vi "Generate Random GB of Size 2015-01-08.vi"() -> ()   [LabVIEW 2010]
uses:
  <vilib>/Utility/file.llb/Write To Spreadsheet File (string).vi
panel:
  out "GBs to Make":cluster{dbl[], dbl[], "Parameter":dbl, dbl[]}[](array[cluster])
  out "# Created":i32
  out "Grain Boundary Definition":T1={"Grain 1 Orientation"=[1.0, 0.8858401549498205, 0.0], "Grain 2 Orientation"=[1.0, 0.3745791306245927, 0.0], "Twist Angle (Deg)"=39.42112887005932, "Translation Vector"=[0.0, 0.0, 0.0]}
  out "Current Index":i32=165102
  out "Status":string="Within range!\nNow creating...\nChecking expected size\nRolling dice...\n"
  in  "Make Random GBs Tab":T2(tab)
  in  "# of Points, Translation":i32
  in  "# of Points, Angle":i32
  in  "# of Points, G2":i32
  in  "Grain 2 or Misorientation Axis":T3={"h, min"=1.0, "h, max"=1.0, "k, min"=0.0, "k, max"=1.0, "l, min"=0.0, "l, max"=1.0} caption="Grain 2 Orientation" {"h, min" format="%#_4f"; "h, max" format="%#_4f"; "k, min" format="%#_4f"; "k, max" format="%#_4f"; "l, min" format="%#_4f"; "l, max" format="%#_4f"}
  in  "Force h>k>l ?":bool=TRUE
  in  "Grain DoF Style":enum32{"Interface-Plane", "Misorientation"}(radio)
  in  "Creation Style":enum32{"Random", "Sequential"}(radio)
  in  "Grain 1 Orientation":T3={"h, min"=1.0, "h, max"=1.0, "k, min"=0.0, "k, max"=1.0, "l, min"=0.0, "l, max"=1.0} {"h, min" format="%#_4f"; "h, max" format="%#_4f"; "k, min" format="%#_4f"; "k, max" format="%#_4f"; "l, min" format="%#_4f"; "l, max" format="%#_4f"}
  in  "Angle Min":dbl caption="Twist Angle"
  in  "Angle Max":dbl=64.0 caption="Max"
  in  "Nearest Integers?":bool
  in  "# to Make":i32
  in  "Translation":T4={"T_x min"=0.0, "T_x max"=3.3, "T_y min"=0.0, "T_y max"=3.3, "T_z min"=0.0, "T_z max"=3.3} {"T_x min" format="%#_4f"; "T_x max" format="%#_4f"; "T_y min" format="%#_4f"; "T_y max" format="%#_4f"; "T_z min" format="%#_4f"; "T_z max" format="%#_4f"}
  in  "# of Points, G1":i32
  out "# of total points":i32
  in  "Max # of Atoms":i32=500
  in  "Require STEM Viewable?":bool
  in  "Number of integers to search":i32=50
  in  "Co-incident Tolerance":dbl=0.01
  in  "Grain Growth and Geometry":T5={"Min Grain Length (A)"=5.0, "Min Angle from GB plane"=0.0, "GB Overlap Length (A)"=0.0}
  in  "Min Seperation Distance (A)":dbl=2.0
  in  "Edge Duplication Range":dbl=3.0
  out "Expected # of atoms":i32=472
  out "# of atoms":i32=2541
  in  "Output Directory":path=path "D:/Ab-initio/RAGB3"
  out "Last Creation Time":T6={"Time to create primitives"=1, "Time to Grow to Box"=5932, "Time to find subset"=6894, "Time to Cleanup"=0}
  out "Structures / Minute":dbl
  in  "Stop Making GBs":bool
  in  "Start Making GBs":bool
  in  "Making GBs":bool
  in  "Conventional Unit Cell":T7={"Structure Name"="CdTe", "Lattice vector a"=[6.615785553057252, 0.0, 0.0], "Lattice vector b"=[0.0, 6.615785553057252, 0.0], "Lattice vector c"=[0.0, 0.0, 6.615785553057252], "Atoms Array"=[{"Atom Name"="Cd", "Positions (Direct)"=[[0.0, 0.0, 0.0], [0.0, 0.5, 0.5], [0.5, 0.0, 0.5], [0.5, 0.5, 0.0]], "Positions (Cartesian)"=[[0.0, 0.0, 0.0], [0.0, 3.307892776528626, 3.307892776528626], [3.307892776528626, 0.0, 3.307892776528626], [3.307892776528626, 3.307892776528626, 0.0]]}, {"Atom Name"="Te", "Positions (Direct)"=[[0.25, 0.25, 0.25], [0.75, 0.75, 0.25], [0.75, 0.25, 0.75], [0.25, 0.75, 0.75]], "Positions (Cartesian)"=[[1.653946388264313, 1.653946388264313, 1.653946388264313], [4.96183916479294, 4.96183916479294, 1.653946388264313], [4.96183916479294, 1.653946388264313, 4.96183916479294], [1.653946388264313, 4.96183916479294, 4.96183916479294]]}], "# of atoms"=8}
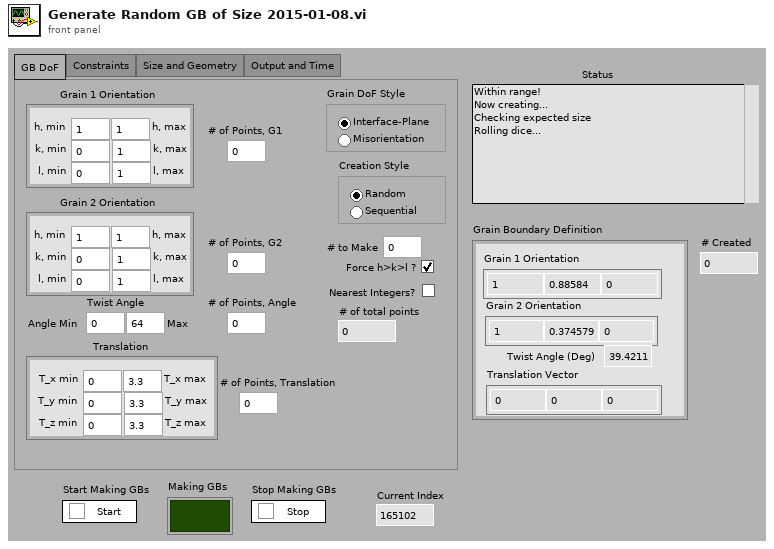
[diagram p1: front panel]
types:
  T1 = cluster{"Grain 1 Orientation":dbl[], "Grain 2 Orientation":dbl[], "Twist Angle (Deg)":dbl, "Translation Vector":dbl[]}
  T2 = enum32{"GB DoF", "Constraints", "Size and Geometry", "Output and Time"}
  T3 = cluster{"h, min":dbl, "h, max":dbl, "k, min":dbl, "k, max":dbl, "l, min":dbl, "l, max":dbl}
  T4 = cluster{"T_x min":dbl, "T_x max":dbl, "T_y min":dbl, "T_y max":dbl, "T_z min":dbl, "T_z max":dbl}
  T5 = cluster{"Min Grain Length (A)":dbl, "Min Angle from GB plane":dbl, "GB Overlap Length (A)":dbl}
  T6 = cluster{"Time to create primitives":u32, "Time to Grow to Box":u32, "Time to find subset":u32, "Time to Cleanup":u32}
  T7 = cluster{"Structure Name":string, "Lattice vector a":dbl[], "Lattice vector b":dbl[], "Lattice vector c":dbl[], "Atoms Array":cluster{"Atom Name":string, "Positions (Direct)":dbl[][], "Positions (Cartesian)":dbl[][]}[], "# of atoms":i32}
  T8 = cluster{dbl[], "Grain 2 Orientation":dbl[], "Twist Angle (Deg)":dbl, dbl[]}
  T9 = cluster{dbl[], "Grain 2 Orientation":dbl[], "Twist Angle (Deg)":dbl}
  T10 = typedef "NI_Matrix.lvlib/RealMatrix.ctl" = dbl[][]
  T11 = cluster{"Misorientation Angle":dbl, "Misorientation Axis, o":dbl[], "Misorientation Matrix":T10}
  T12 = cluster{"h, min":dbl, "h, max":dbl, "# of Points, G1":i32}
  T13 = cluster{"k, min":dbl, "k, max":dbl, "# of Points, G1":i32}
  T14 = cluster{"l, min":dbl, "l, max":dbl, "# of Points, G1":i32}
  T15 = cluster{"h, min":dbl, "h, max":dbl, "# of Points, G2":i32}
  T16 = cluster{"k, min":dbl, "k, max":dbl, "# of Points, G2":i32}
  T17 = cluster{"l, min":dbl, "l, max":dbl, "# of Points, G2":i32}
  T18 = cluster{"Angle Min":dbl, "Angle Max":dbl, "# of Points, Angle":i32}
  T19 = cluster{"T_x min":dbl, "T_x max":dbl, "# of Points, Translation":i32}
  T20 = cluster{"T_y min":dbl, "T_y max":dbl, "# of Points, Translation":i32}
  T21 = cluster{"T_z min":dbl, "T_z max":dbl, "# of Points, Translation":i32}
  T22 = cluster{"T_z min":dbl, "T_z max":dbl, "# of Points, Translation":i32}[]
  T23 = cluster{"T_z min":dbl, "T_z max":dbl, "# of Points, Translation":i32, "Style":enum16{"Linear Step", "Linear Pts", "Log Pts"}, string}
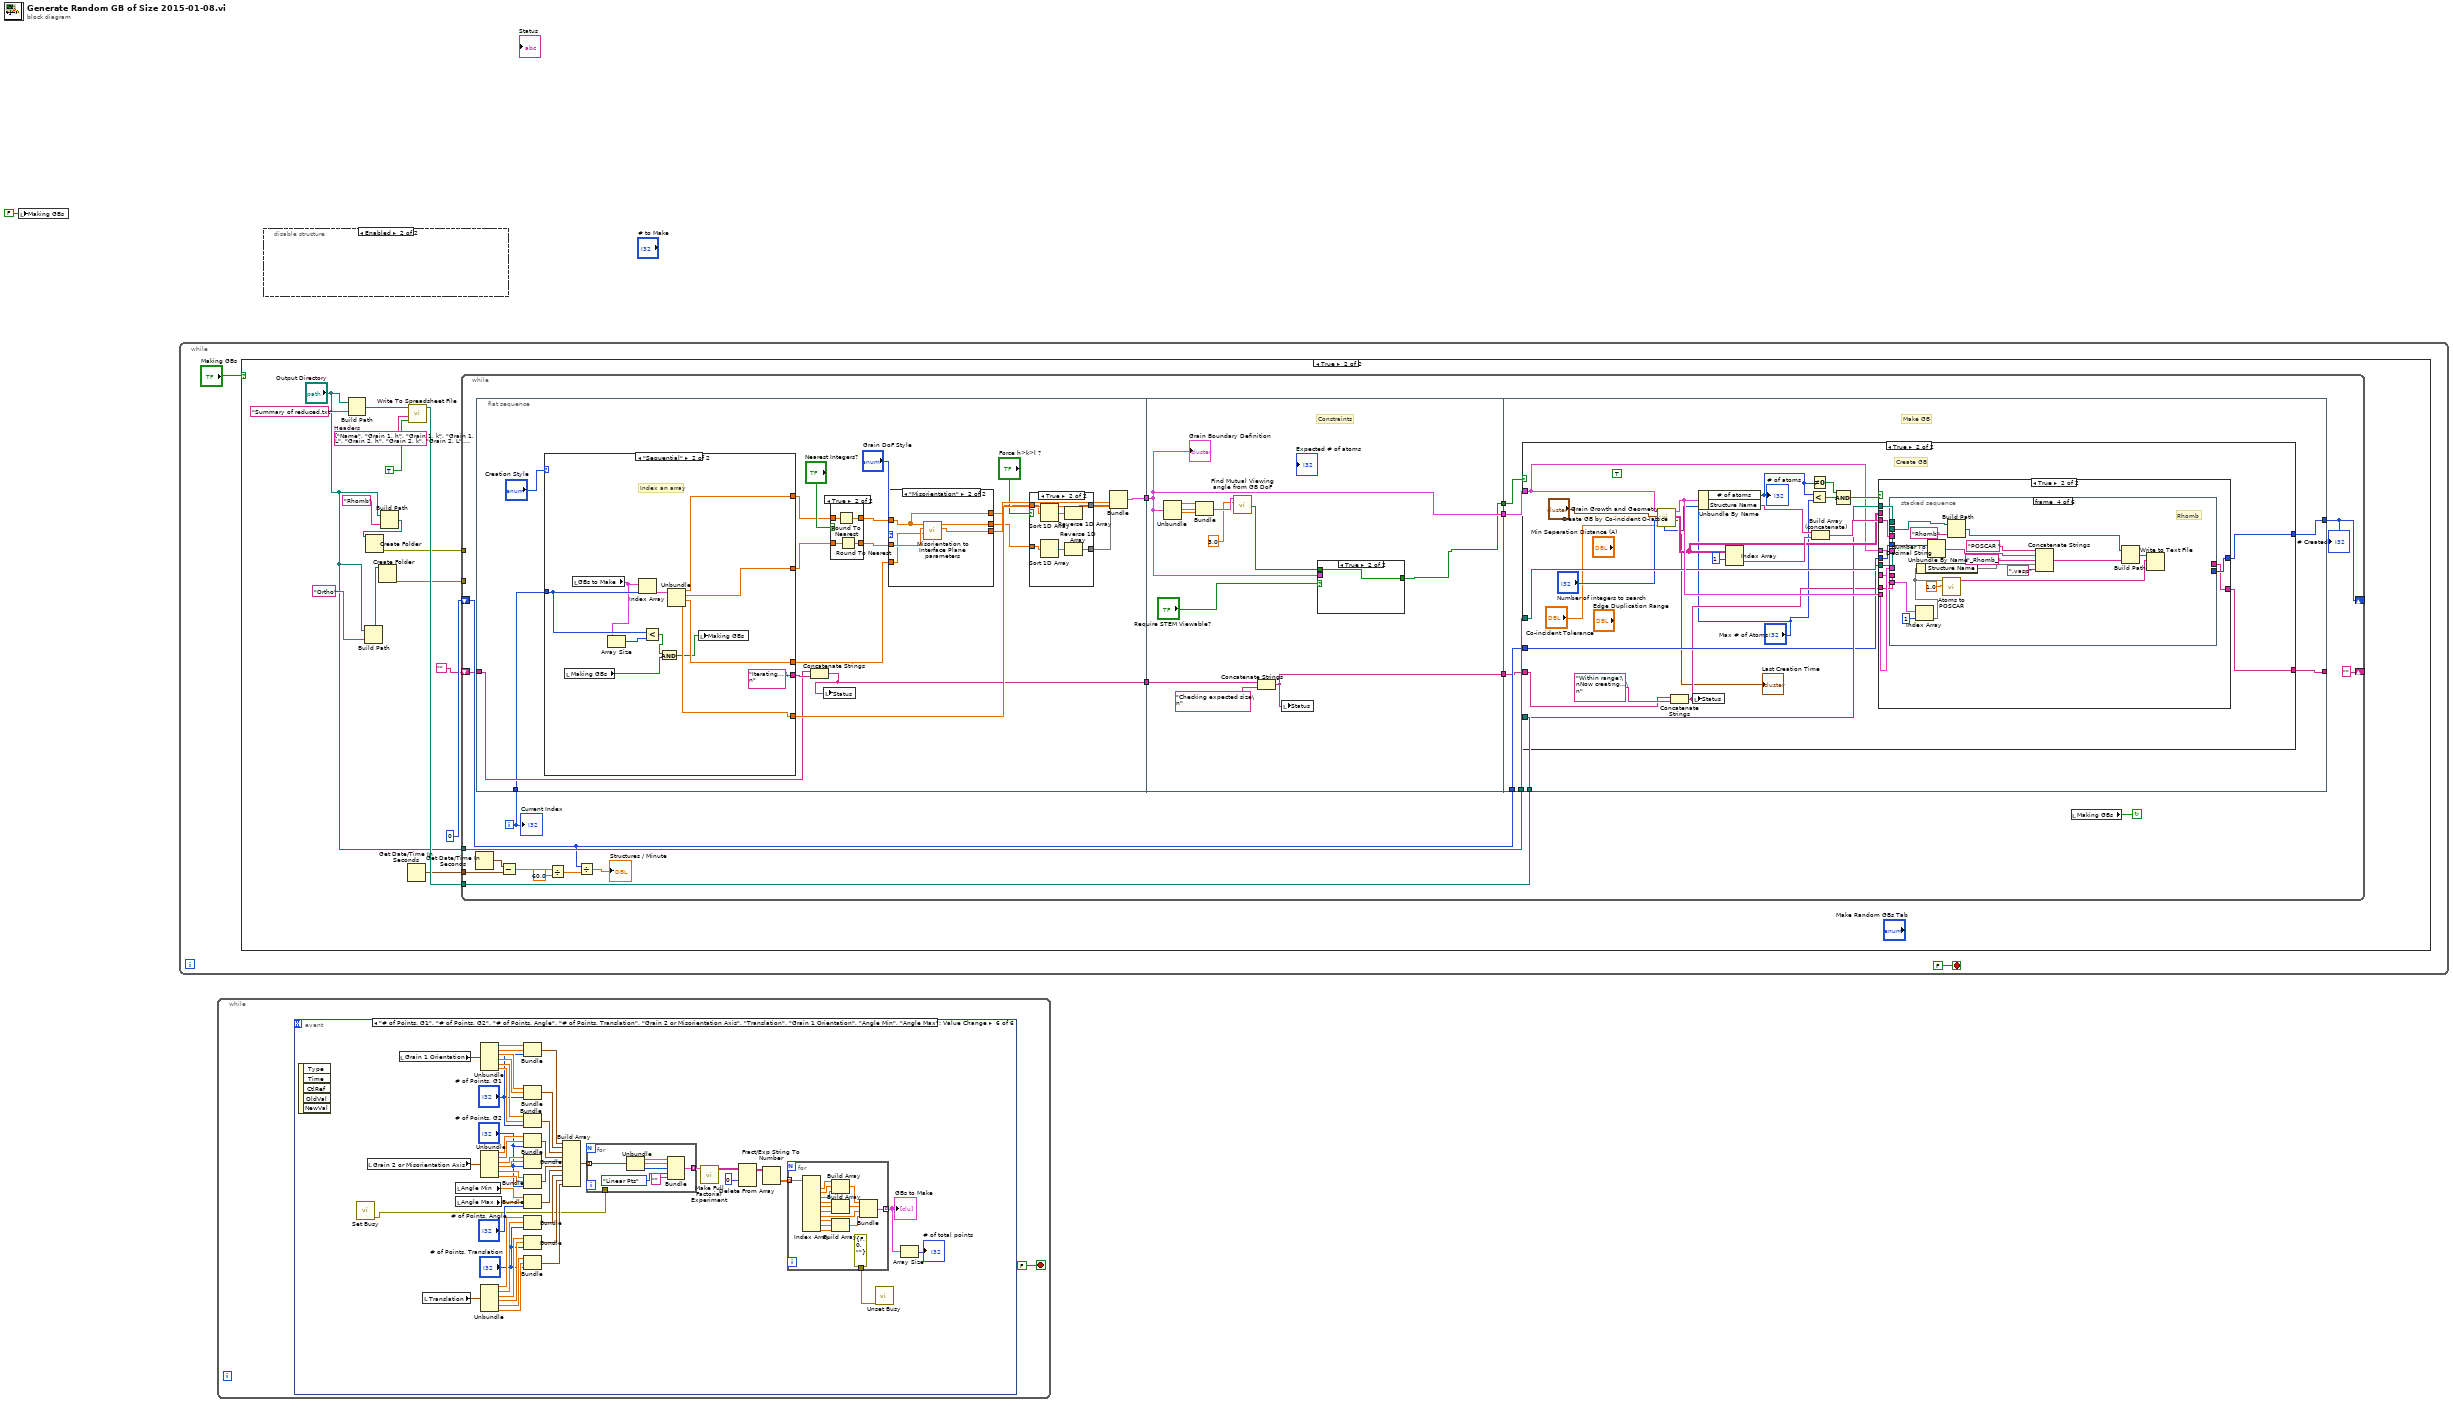
[diagram p0: block diagram]
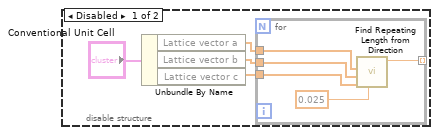
[diagram p2: hidden frame]
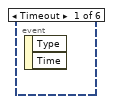
[diagram p3: hidden frame]
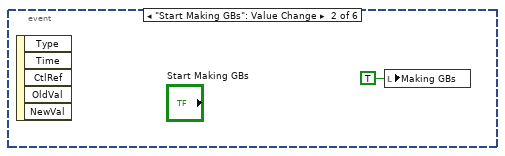
[diagram p4: hidden frame]
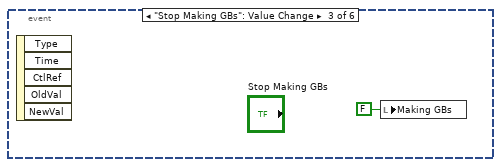
[diagram p5: hidden frame]
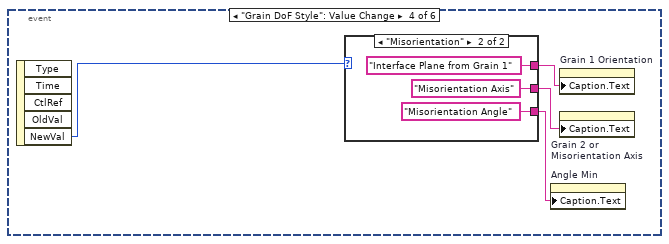
[diagram p6: hidden frame]
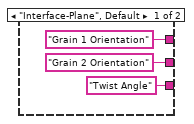
[diagram p7: hidden frame]
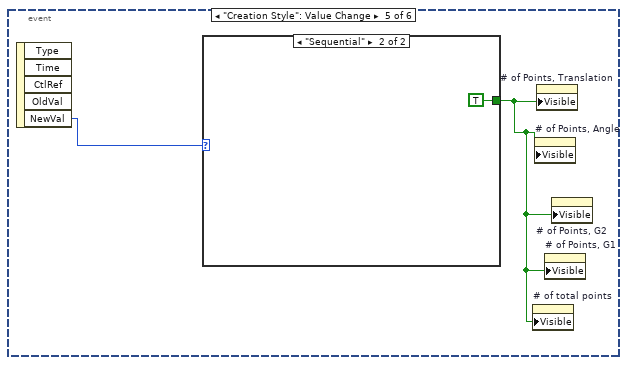
[diagram p8: hidden frame]
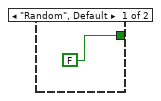
[diagram p9: hidden frame]
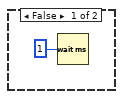
[diagram p10: hidden frame]
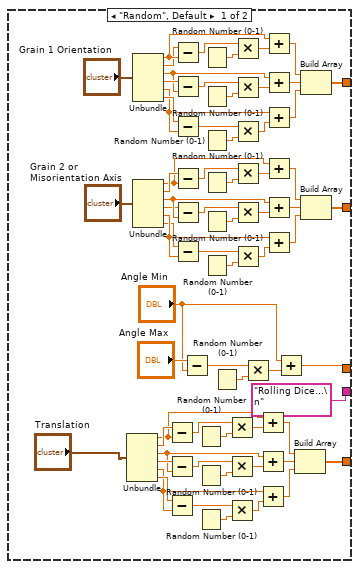
[diagram p14: hidden frame]
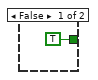
[diagram p15: hidden frame]
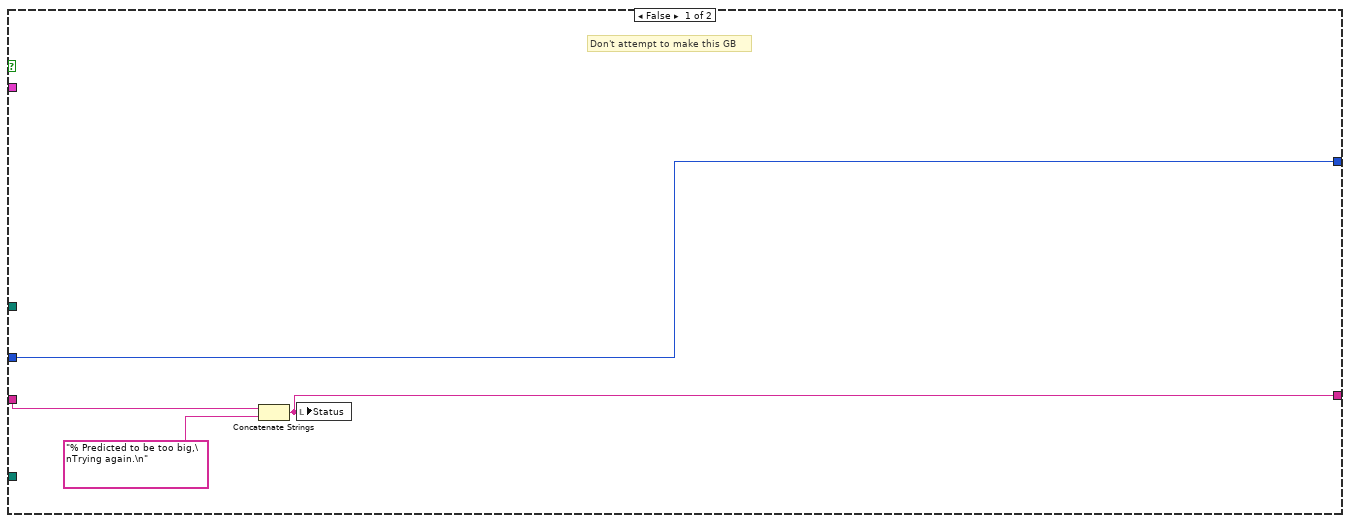
[diagram p16: hidden frame]
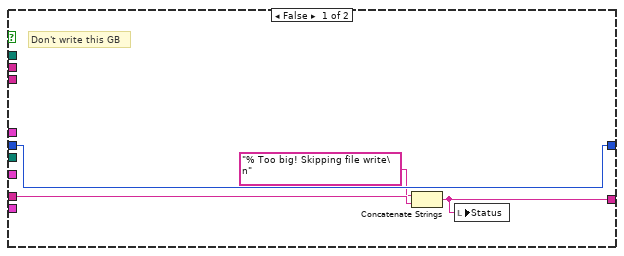
[diagram p17: hidden frame]
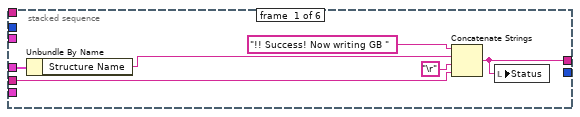
[diagram p18: hidden frame]
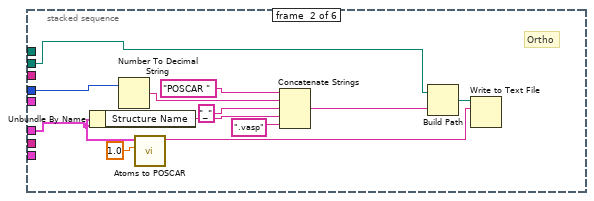
[diagram p19: hidden frame]
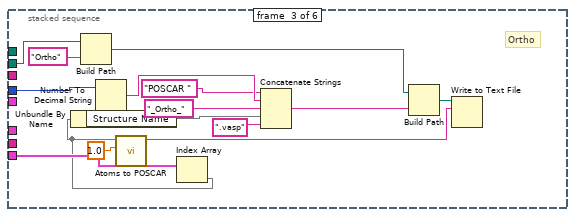
[diagram p20: hidden frame]
diagram:
  n1 = local write "Making GBs"(FALSE ("Making GBs")) -> ()
  n2 = while {
    stop <- FALSE stop-if-true
    n3 = case shown="True" "Making GBs" {
      frame False {
        n4 = Wait (ms)(milliseconds to wait=u32 1) -> ()  [unwired: 1 out]
      }
      frame True {
        w16 = string[] ["Name", "Grain 1, h", "Grain 1, k", "Grain 1, L", "Grain 2, h", "Grain 2, k", "Grain 2, L", "Twist Angle (Deg)", "Translation Tx", "Translation Ty", "Translation Tz", "Tilt Angle (Deg)", "Viewing Angle, h", "Viewing Angle, k", "Viewing Angle, L", "Grain 1 Length (factor)", "Grain 2 Length (factor", "Max Grain Height (A)", "Max Grain Width (A)", "Grain 1 Start", "Overlap Region (A)", "Reduction Slab X", "Reduction Slab Y", "Reduction Tolerance (A)", "Min Atomic Separation Distance", "Edge Duplication Range", "# of Atoms", "STEM Direction,h", "STEM Direction,k", "STEM Direction,l", "Grain 1, [h]", "Grain 1, [k]", "Grain 1, [L]", "Grain 2, [h]", "Grain 2, [k]", "Grain 2, [L]", "Misorientaton Angle (Deg)", "Misorientation Axis, h", "Misorientation Axis, k", "Misorientation Axis, l"]  # Headers
        n5 = Build Path(base path="Output Directory", name or relative path="Summary of reduced.txt") -> (appended path=w17:path)
        n6 = Build Path(base path="Output Directory", name or relative path="Ortho") -> (appended path=w8:path)
        n7 = Create Folder(path (use dialog)=w8) -> (error out=w6:errorcluster)  [unwired: 2 in, 2 out]
        n8 = Build Path(base path="Output Directory", name or relative path="Rhomb") -> (appended path=w10:path)
        n9 = Create Folder(path (use dialog)=w10) -> (error out=w7:errorcluster)  [unwired: 2 in, 2 out]
        n10 = Get Date/Time In Seconds() -> (seconds since 1Jan1904=w12:timestamp)
        n11 = call-poly <vilib>:"Write To Spreadsheet File.vi"("append to file? (new file:F)"=TRUE, "1D data"=w16, "file path (dialog if empty)"=w17) -> ("new file path (Not A Path if cancelled)"=w14:path)  [unwired: 5 in]
        n12 = while {
          shift-right: [w28] -> _
          shift-left: 0 -> [w29]
          tunnel: w12 -> [w35]
          tunnel: "Output Directory" -> [w31]
          tunnel: w14 -> [w30]
          shift-right: [""] -> _
          shift-left: "" -> [w27]
          tunnel: w7 -> [_]
          tunnel: w6 -> [_]
          i -> [w20]
          stop <- w25 continue-if-true
          n13 = Get Date/Time In Seconds() -> (seconds since 1Jan1904=w23:timestamp)
          n14 = flat-sequence {
            tunnel: w27 -> [w40]
            tunnel: [w43] -> w22
            tunnel: [w41] -> w21
            tunnel: w20 -> [w39]
            tunnel: [w168] -> w33
            tunnel: [w160] -> w32
            tunnel: [w170] -> w26
            tunnel: w22 -> [w168]
            tunnel: w21 -> [w163]
            tunnel: w33 -> [w177]
            tunnel: w32 -> [w181]
            tunnel: w31 -> [w180]
            tunnel: w30 -> [w179]
            tunnel: w29 -> [w178]
            tunnel: [w176] -> w28
            tunnel: w26 -> [w175]
            tunnel: [w174] -> _
            frame #0 {
              n15 = case shown="\"Sequential\"" "Creation Style" {
                tunnel: [w110 w157] -> w45
                tunnel: [w109 w156] -> w46
                tunnel: [w103 w155] -> w51
                tunnel: [w84 w154] -> w58
                tunnel: ["Rolling Dice...\n" ("string") "Iterating... \n" ("string")] -> w42
                tunnel: w39 -> [_ w153]
                frame "Random", Default {
                  n16 = Unbundle("Translation") -> ("T_x min"=w82:dbl, "T_x max"=w86:dbl, "T_y min"=w93:dbl, "T_y max"=w94:dbl, "T_z min"=w95:dbl, "T_z max"=w96:dbl)
                  n17 = Unbundle("Grain 1 Orientation") -> ("h, min"=w136:dbl, "h, max"=w133:dbl, "k, min"=w141:dbl, "k, max"=w142:dbl, "l, min"=w143:dbl, "l, max"=w144:dbl)
                  n18 = Unbundle("Grain 2 or Misorientation Axis") -> ("h, min"=w83:dbl, "h, max"=w131:dbl, "k, min"=w124:dbl, "k, max"=w123:dbl, "l, min"=w122:dbl, "l, max"=w121:dbl)
                  n19 = Subtract(x=w86, y=w82) -> (x-y=w87:dbl)
                  n20 = Subtract(x=w94, y=w93) -> (x-y=w90:dbl)
                  n21 = Subtract(x=w96, y=w95) -> (x-y=w91:dbl)
                  n22 = Subtract(x=w133, y=w136) -> (x-y=w134:dbl)
                  n23 = Subtract(x=w142, y=w141) -> (x-y=w138:dbl)
                  n24 = Subtract(x=w144, y=w143) -> (x-y=w139:dbl)
                  n25 = Subtract(x=w131, y=w83) -> (x-y=w130:dbl)
                  n26 = Subtract(x=w123, y=w124) -> (x-y=w127:dbl)
                  n27 = Subtract(x=w121, y=w122) -> (x-y=w126:dbl)
                  n28 = Subtract(x="Angle Max", y="Angle Min") -> (x-y=w106:dbl)
                  n29 = Random Number (0-1)() -> (number: 0 to 1=w97:dbl)
                  n30 = Random Number (0-1)() -> (number: 0 to 1=w98:dbl)
                  n31 = Random Number (0-1)() -> (number: 0 to 1=w99:dbl)
                  n32 = Random Number (0-1)() -> (number: 0 to 1=w145:dbl)
                  n33 = Random Number (0-1)() -> (number: 0 to 1=w146:dbl)
                  n34 = Random Number (0-1)() -> (number: 0 to 1=w147:dbl)
                  n35 = Random Number (0-1)() -> (number: 0 to 1=w120:dbl)
                  n36 = Random Number (0-1)() -> (number: 0 to 1=w119:dbl)
                  n37 = Random Number (0-1)() -> (number: 0 to 1=w118:dbl)
                  n38 = Random Number (0-1)() -> (number: 0 to 1=w108:dbl)
                  n39 = Multiply(x=w87, y=w97) -> (x*y=w88:dbl)
                  n40 = Multiply(x=w90, y=w98) -> (x*y=w89:dbl)
                  n41 = Multiply(x=w91, y=w99) -> (x*y=w92:dbl)
                  n42 = Multiply(x=w134, y=w145) -> (x*y=w135:dbl)
                  n43 = Multiply(x=w138, y=w146) -> (x*y=w137:dbl)
                  n44 = Multiply(x=w139, y=w147) -> (x*y=w140:dbl)
                  n45 = Multiply(x=w130, y=w120) -> (x*y=w129:dbl)
                  n46 = Multiply(x=w127, y=w119) -> (x*y=w128:dbl)
                  n47 = Multiply(x=w126, y=w118) -> (x*y=w125:dbl)
                  n48 = Multiply(x=w106, y=w108) -> (x*y=w107:dbl)
                  n49 = Add(x=w82, y=w88) -> (x+y=w100:dbl)
                  n50 = Add(x=w93, y=w89) -> (x+y=w101:dbl)
                  n51 = Add(x=w95, y=w92) -> (x+y=w102:dbl)
                  n52 = Add(x=w136, y=w135) -> (x+y=w116:dbl)
                  n53 = Add(x=w141, y=w137) -> (x+y=w115:dbl)
                  n54 = Add(x=w143, y=w140) -> (x+y=w114:dbl)
                  n55 = Add(x=w83, y=w129) -> (x+y=w113:dbl)
                  n56 = Add(x=w124, y=w128) -> (x+y=w112:dbl)
                  n57 = Add(x=w122, y=w125) -> (x+y=w111:dbl)
                  n58 = Add(x="Angle Min", y=w107) -> (x+y=w103:dbl)
                  n59 = Build Array(w100, w101, w102) -> (w84:dbl[])
                  n60 = Build Array(w116, w115, w114) -> (w110:dbl[])
                  n61 = Build Array(w113, w112, w111) -> (w109:dbl[])
                }
                frame "Sequential" {
                  # "Index an array"
                  n62 = local read "Making GBs"() -> (w149:bool)
                  n63 = local read "GBs to Make"() -> (w152:cluster{dbl[], dbl[], "Parameter":dbl, dbl[]}[])
                  n64 = Array Size(array=w152) -> (size(s)=w151:i32)
                  n65 = Index Array(array=w152, index=w153) -> (element=w158:cluster{dbl[], dbl[], "Parameter":dbl, dbl[]})
                  n66 = Less?(x=w153, y=w151) -> (x < y?=w150:bool)
                  n67 = And(x=w150, y=w149) -> (x .and. y?=w148:bool)
                  n68 = Unbundle(w158) -> (w157:dbl[], w156:dbl[], "Parameter"=w155:dbl, w154:dbl[])
                  n69 = local write "Making GBs"(w148) -> ()
                }
              }
              n70 = Concatenate Strings(w40, w42) -> (w41:string)
              n71 = local write "Status"(w41) -> ()
              n72 = case shown="True" "Nearest Integers?" {
                tunnel: [w75 w80] -> w50
                tunnel: [w76 w79] -> w49
                tunnel: w45 -> [w76 w78]
                tunnel: w46 -> [w75 w77]
                frame False {
                }
                frame True {
                  n73 = Round To Nearest(number=w78) -> (nearest integer value=w79:dbl[])
                  n74 = Round To Nearest(number=w77) -> (nearest integer value=w80:dbl[])
                }
              }
              n75 = case shown="\"Misorientation\"" "Grain DoF Style" {
                tunnel: w49 -> [w69 w71]
                tunnel: w50 -> [w68 w74]
                tunnel: w51 -> [w67 w73]
                tunnel: [w68 w72] -> w54
                tunnel: [w69 w71] -> w52
                tunnel: [w67 w70] -> w57
                frame "Interface-Plane", Default {
                }
                frame "Misorientation" {
                  n76 = call "Misorientation to Interface Plane parameters.vi"("Misorientation Angle"=w73, "Misorientation Axis, o"=w74, "Grain 1 Orientation"=w71) -> ("Twist Angle (Deg)"=w70:dbl, "Grain 2 Orientation"=w72:dbl[])  [unwired: 5 in, 2 out]
                }
              }
              n77 = case shown="True" "Force h>k>l ?" {
                tunnel: [w60 w64] -> w55
                tunnel: w52 -> [w60 w66]
                tunnel: w54 -> [w59 w62]
                tunnel: [w59 w61] -> w56
                frame False {
                }
                frame True {
                  n78 = Sort 1D Array(array=w66) -> (sorted array=w65:dbl[])
                  n79 = Sort 1D Array(array=w62) -> (sorted array=w63:dbl[])
                  n80 = Reverse 1D Array(array=w65) -> (reversed array=w64:dbl[])
                  n81 = Reverse 1D Array(array=w63) -> (reversed array=w61:dbl[])
                }
              }
              n82 = Bundle(w55, "Grain 2 Orientation"=w56, "Twist Angle (Deg)"=w57, w58) -> (w43:T8)  [unwired: 1 in]
            }
            frame #1 {
              # "Constraints"
              n83 = Unbundle(w168) -> (w167:dbl[], "Grain 2 Orientation"=w166:dbl[], "Twist Angle (Deg)"=w165:dbl)  [unwired: 1 out]
              n84 = Bundle(w167, "Grain 2 Orientation"=w166, "Twist Angle (Deg)"=w165) -> (w164:T9)  [unwired: 1 in]
              n85 = call "Find Mutual Viewing angle from GB DoF.vi"("Viewing Angle Tolerance (Deg)"=3.0 ("Integer Tolerance"), "Grain Boundary Macro DoF"=w164) -> ("STEM Viewable?"=w161:bool)  [unwired: 7 in, 2 out]
              n86 = Concatenate Strings(w163, "Checking expected size\n" ("string")) -> (w170:string)
              n87 = local write "Status"(w170) -> ()
              n88 = case shown="True" "Require STEM Viewable?" {
                tunnel: w168 -> [_ _]
                tunnel: [TRUE ("STEM Viewable?") w173] -> w160
                tunnel: w161 -> [_ w173]
                frame False {
                }
                frame True {
                }
              }
              "Grain Boundary Definition" <- w168
            }
            frame #2 {
              # "Make GB"
              n89 = case shown="True" w181 {
                tunnel: w180 -> [_ w205]
                tunnel: w179 -> [_ w204]
                tunnel: w178 -> [w185 w203]
                tunnel: w177 -> [_ w192]
                tunnel: [w185 w197] -> w176
                tunnel: w175 -> [w184 w195]
                tunnel: [w182 w193] -> w174
                frame False {
                  # "Don't attempt to make this GB"
                  n90 = Concatenate Strings(w184, "% Predicted to be too big,\nTrying again.\n" ("string")) -> (w182:string)
                  n91 = local write "Status"(w182) -> ()
                }
                frame True {
                  w202 = TRUE ("Skip cleanup if no subset")
                  # "Create GB"
                  n92 = call "Create GB by Co-incident O-lattice.vi"("Max # of atoms"="Max # of Atoms", "Co-incident Tolerance"="Co-incident Tolerance", "Number of integers to search"="Number of integers to search", "Grain Growth and Geometry"="Grain Growth and Geometry", "Grain Boundary Definition"=w192) -> ("Creation Time"=→"Last Creation Time":T6, "GB Data"=w208:string[][], "Grain Boundary"=w209:T7)  [unwired: 4 in]
                  n93 = Concatenate Strings(w195, "Within range!\nNow creating...\n" ("string")) -> (w194:string)
                  n94 = local write "Status"(w194) -> ()
                  n95 = Unbundle By Name(w209) -> ("# of atoms"=w201:i32, "Structure Name"=w213:string)
                  "# of atoms" <- w201
                  n96 = Index Array(array=w208, index (row)=1) -> (element=w211:string[])  [unwired: 1 in]
                  n97 = Less?(x=w201, y="Max # of Atoms") -> (x < y?=w199:bool)
                  n98 = Not Equal To 0?(x=w201) -> (x != 0?=w200:bool)
                  n99 = Build Array (concatenate)(w213, w211) -> (w212:string[])
                  n100 = Compound Arithmetic op=AND(w200, w199) -> (w198:bool)  [unwired: 1 in]
                  n101 = case shown="True" w198 {
                    tunnel: w203 -> [w217 w225]
                    tunnel: [w217 w224] -> w197
                    tunnel: w208 -> [_ _]
                    tunnel: w209 -> [_ w227]
                    tunnel: w212 -> [_ w222]
                    tunnel: w205 -> [_ w226]
                    tunnel: w204 -> [_ w223]
                    tunnel: w194 -> [w216 w220]
                    tunnel: [w215 w219] -> w193
                    tunnel: w192 -> [_ w221]
                    tunnel: [_ w218] -> w191
                    frame False {
                      # "Don't write this GB"
                      n102 = Concatenate Strings("% Too big! Skipping file write\n" ("string"), w216) -> (w215:string)
                      n103 = local write "Status"(w215) -> ()
                    }
                    frame True {
                      n104 = stacked-sequence {
                        tunnel: w227 -> [w231 w234 _ _ _ _]
                        tunnel: w226 -> [_ w235 w249 w263 _ _]
                        tunnel: w225 -> [_ w241 w256 w272 w278 _]
                        tunnel: [_ _ _ _ w277 _] -> w224
                        tunnel: w223 -> [_ _ _ _ _ w292]
                        tunnel: w222 -> [_ _ _ _ _ w290]
                        tunnel: w221 -> [_ _ _ _ _ w284]
                        tunnel: w220 -> [w229 _ _ _ _ _]
                        tunnel: [w228 _ _ _ _ _] -> w219
                        tunnel: w218 -> [_ _ w247 w266 _ _]
                        frame #0 {
                          n105 = Unbundle By Name(w231) -> ("Structure Name"=w230:string)
                          n106 = Concatenate Strings("!! Success! Now writing GB " ("string"), w230, "\r", w229) -> (w228:string)
                          n107 = local write "Status"(w228) -> ()
                        }
                        frame #1 {
                          # "Ortho"
                          n108 = Unbundle By Name(w234) -> ("Structure Name"=w238:string)
                          n109 = Number To Decimal String(number=w241) -> (decimal integer string=w245:string)  [unwired: 1 in]
                          n110 = call "Atoms to POSCAR.vi"("Volume Factor"=1.0, "Atomic Structure"=w234) -> ("POSCAR File"=w240:string)  [unwired: 9 in]
                          n111 = Concatenate Strings("POSCAR " ("string"), w245, "_" ("string"), w238, ".vasp" ("string")) -> (w244:string)
                          n112 = Build Path(base path=w235, name or relative path=w244) -> (appended path=w236:path)
                          n113 = Write to Text File(file (use dialog)=w236, text=w240) -> ()  [unwired: 2 in, 3 out]
                        }
                        frame #2 {
                          # "Ortho"
                          n114 = Build Path(base path=w249, name or relative path="Ortho") -> (appended path=w248:path)
                          n115 = Number To Decimal String(number=w256) -> (decimal integer string=w260:string)  [unwired: 1 in]
                          n116 = Index Array(array=w247) -> (element=w246)  [unwired: 1 in]
                          n117 = Unbundle By Name(w246) -> ("Structure Name"=w253)
                          n118 = call "Atoms to POSCAR.vi"("Volume Factor"=1.0, "Atomic Structure"=w246) -> ("POSCAR File"=w255:string)  [unwired: 9 in]
                          n119 = Concatenate Strings("POSCAR " ("string"), w260, "_Ortho_" ("string"), w253, ".vasp" ("string")) -> (w259:string)
                          n120 = Build Path(base path=w248, name or relative path=w259) -> (appended path=w251:path)
                          n121 = Write to Text File(file (use dialog)=w251, text=w255) -> ()  [unwired: 2 in, 3 out]
                        }
                        frame #3 {
                          # "Rhomb"
                          n122 = Index Array(array=w266, index=1) -> (element=w264)
                          n123 = Unbundle By Name(w264) -> ("Structure Name"=w269)
                          n124 = Number To Decimal String(number=w272) -> (decimal integer string=w276:string)  [unwired: 1 in]
                          n125 = call "Atoms to POSCAR.vi"("Volume Factor"=1.0, "Atomic Structure"=w264) -> ("POSCAR File"=w271:string)  [unwired: 9 in]
                          n126 = Build Path(base path=w263, name or relative path="Rhomb") -> (appended path=w262:path)
                          n127 = Concatenate Strings("POSCAR " ("string"), w276, "_Rhomb_" ("string"), w269, ".vasp" ("string")) -> (w275:string)
                          n128 = Build Path(base path=w262, name or relative path=w275) -> (appended path=w267:path)
                          n129 = Write to Text File(file (use dialog)=w267, text=w271) -> ()  [unwired: 2 in, 3 out]
                        }
                        frame #4 {
                          n130 = Increment(x=w278) -> (x+1=w277:i32)
                        }
                        frame #5 {
                          n131 = call "Analyze GB - Detail.vi"("Find Integer Rep?"=TRUE, "Grain Boundary Definition"=w284) -> ("Misorientation"=w288:T11, "Grain 2 Integers"=w287:dbl[], "Grain 1 Integers"=w286:dbl[], "Suggested view direction"=w279:dbl[])  [unwired: 2 in, 4 out]
                          n132 = Unbundle By Name(w288) -> ("Misorientation Angle"=w283:dbl, "Misorientation Axis, o"=w282:dbl[])
                          n133 = Build Array (concatenate)(w279, w286, w287, w283, w282) -> (w281:dbl[])
                          n134 = Number To Fractional String(number=w281) -> (F-format string=w280:string[])  [unwired: 3 in]
                          n135 = Build Array (concatenate)(w290, w280) -> (w289:string[])
                          n136 = call-poly <vilib>:"Write To Spreadsheet File.vi"("append to file? (new file:F)"=TRUE, "1D data"=w289, "file path (dialog if empty)"=w292) -> ()  [unwired: 5 in, 1 out]
                        }
                      }
                    }
                  }
                }
              }
            }
          }
          n137 = Subtract(x=w23, y=w35) -> (x-y=w37:dbl)
          n138 = Divide(x=w37, y=60.0) -> (x/y=w34:dbl)
          n139 = Divide(x=w29, y=w34) -> (x/y=→"Structures / Minute":dbl)
          n140 = local read "Making GBs"() -> (w25:bool)
          "Current Index" <- w20
          "# Created" <- w28
        }
      }
    }
  }
  n141 = while {
    stop <- FALSE stop-if-true
    n142 = event shown="[5] \"# of Points, G1\", \"# of Points, G2\", \"# of Points, Angle\", \"# of Points, Translation\", \"Grain 2 or Misorientation Axis\", \"Translation\", \"Grain 1 Orientation\", \"Angle Min\", \"Angle Max\": Value Change" {
      selector: _ -> [_ _ _ _ _ _]
      dyn-events: _ -> [_ _ _ _ _ _]
      timeout: _ -> [_ _ _ _ _ _]
      event Timeout {
        n143 = event-data() -> ()  [unwired: 1 in, 2 out]
      }
      event "Start Making GBs": Value Change {
        n144 = event-data() -> ()  [unwired: 1 in, 5 out]
        n145 = local write "Making GBs"(TRUE ("Making GBs")) -> ()
      }
      event "Stop Making GBs": Value Change {
        n146 = event-data() -> ()  [unwired: 1 in, 5 out]
        n147 = local write "Making GBs"(FALSE ("Making GBs")) -> ()
      }
      event "Grain DoF Style": Value Change {
        n148 = event-data() -> ("NewVal"=w299:enum32{"Interface-Plane", "Misorientation"})  [unwired: 1 in, 4 out]
        n149 = case shown="\"Misorientation\"" w299 {
          tunnel: ["Grain 1 Orientation" ("Caption.Text") "Interface Plane from Grain 1" ("Caption.Text")] -> w298
          tunnel: ["Grain 2 Orientation" ("Caption.Text") "Misorientation Axis" ("Caption.Text")] -> w297
          tunnel: ["Twist Angle" ("Caption.Text") "Misorientation Angle" ("Caption.Text")] -> w296
          frame "Interface-Plane", Default {
          }
          frame "Misorientation" {
          }
        }
        n150 = property on="Angle Min" class="DigNum (strict)"("Caption.Text"=w296) -> ()  [unwired: 2 in, 2 out]
        n151 = property on="Grain 1 Orientation" class="Clust (strict)"("Caption.Text"=w298) -> ()  [unwired: 2 in, 2 out]
        n152 = property on="Grain 2 or Misorientation Axis" class="Clust (strict)"("Caption.Text"=w297) -> ()  [unwired: 2 in, 2 out]
      }
      event "Creation Style": Value Change {
        n153 = event-data() -> ("NewVal"=w307:enum32{"Random", "Sequential"})  [unwired: 1 in, 4 out]
        n154 = case shown="\"Sequential\"" w307 {
          tunnel: [FALSE ("Visible") TRUE ("Visible")] -> w306
          frame "Random", Default {
          }
          frame "Sequential" {
          }
        }
        n155 = property on="# of total points" class="DigNum (strict)"("Visible"=w306) -> ()  [unwired: 2 in, 2 out]
        n156 = property on="# of Points, Angle" class="DigNum (strict)"("Visible"=w306) -> ()  [unwired: 2 in, 2 out]
        n157 = property on="# of Points, Translation" class="DigNum (strict)"("Visible"=w306) -> ()  [unwired: 2 in, 2 out]
        n158 = property on="# of Points, G1" class="DigNum (strict)"("Visible"=w306) -> ()  [unwired: 2 in, 2 out]
        n159 = property on="# of Points, G2" class="DigNum (strict)"("Visible"=w306) -> ()  [unwired: 2 in, 2 out]
      }
      event "# of Points, G1", "# of Points, G2", "# of Points, Angle", "# of Points, Translation", "Grain 2 or Misorientation Axis", "Translation", "Grain 1 Orientation", "Angle Min", "Angle Max": Value Change {
        n160 = event-data() -> ()  [unwired: 1 in, 5 out]
        n161 = call <vilib>:"Set Busy.vi"() -> ("error out"=w311:errorcluster)  [unwired: 10 in, 1 out]
        n162 = local read "Grain 2 or Misorientation Axis"() -> (w343:T3)
        n163 = local read "Grain 1 Orientation"() -> (w356:T3)
        n164 = local read "Translation"() -> (w334:T4)
        n165 = local read "Angle Min"() -> (w333:dbl)
        n166 = local read "Angle Max"() -> (w332:dbl)
        n167 = Unbundle(w356) -> ("h, min"=w355:dbl, "h, max"=w354:dbl, "k, min"=w353:dbl, "k, max"=w352:dbl, "l, min"=w351:dbl, "l, max"=w350:dbl)
        n168 = Unbundle(w343) -> ("h, min"=w344:dbl, "h, max"=w345:dbl, "k, min"=w346:dbl, "k, max"=w347:dbl, "l, min"=w348:dbl, "l, max"=w349:dbl)
        n169 = Unbundle(w334) -> ("T_x min"=w340:dbl, "T_x max"=w339:dbl, "T_y min"=w338:dbl, "T_y max"=w337:dbl, "T_z min"=w336:dbl, "T_z max"=w335:dbl)
        n170 = Bundle("h, min"=w355, "h, max"=w354, "# of Points, G1"="# of Points, G1") -> (w329:T12)  [unwired: 1 in]
        n171 = Bundle("k, min"=w353, "k, max"=w352, "# of Points, G1"="# of Points, G1") -> (w328:T13)  [unwired: 1 in]
        n172 = Bundle("l, min"=w351, "l, max"=w350, "# of Points, G1"="# of Points, G1") -> (w327:T14)  [unwired: 1 in]
        n173 = Bundle("h, min"=w344, "h, max"=w345, "# of Points, G2"="# of Points, G2") -> (w326:T15)  [unwired: 1 in]
        n174 = Bundle("k, min"=w346, "k, max"=w347, "# of Points, G2"="# of Points, G2") -> (w325:T16)  [unwired: 1 in]
        n175 = Bundle("l, min"=w348, "l, max"=w349, "# of Points, G2"="# of Points, G2") -> (w324:T17)  [unwired: 1 in]
        n176 = Bundle("Angle Min"=w333, "Angle Max"=w332, "# of Points, Angle"="# of Points, Angle") -> (w323:T18)  [unwired: 1 in]
        n177 = Bundle("T_x min"=w340, "T_x max"=w339, "# of Points, Translation"="# of Points, Translation") -> (w322:T19)  [unwired: 1 in]
        n178 = Bundle("T_y min"=w338, "T_y max"=w337, "# of Points, Translation"="# of Points, Translation") -> (w321:T20)  [unwired: 1 in]
        n179 = Bundle("T_z min"=w336, "T_z max"=w335, "# of Points, Translation"="# of Points, Translation") -> (w320:T21)  [unwired: 1 in]
        n180 = Build Array(w329, w328, w327, w326, w325, w324, w323, w322, w321, w320) -> (w319:T22)
        n181 = for {
          tunnel: w319 -> [w379] mode=indexing
          tunnel: [w374] -> w318 mode=indexing
          tunnel: w311 -> [_]
          n182 = Unbundle(w379) -> ("T_z min"=w378:dbl, "T_z max"=w377:dbl, "# of Points, Translation"=w376:i32)
          n183 = Bundle("T_z min"=w378, "T_z max"=w377, "# of Points, Translation"=w376, "Style"=enum16{"Linear Step", "Linear Pts", "Log Pts"}."Linear Pts", "") -> (w374:T23)  [unwired: 1 in]
        }
        n184 = call "Make Full Factorial Experiment.vi"("Array of Array Settings"=w318) -> ("Full Factorial Design"=w317:string[][])  [unwired: 10 in]
        n185 = Delete From Array(array=w317, index (row)=0) -> (array with subset deleted=w315:string[][])  [unwired: 2 in, 1 out]
        n186 = Fract/Exp String To Number(string=w315) -> (number=w314:dbl[][])  [unwired: 3 in, 1 out]
        n187 = for {
          tunnel: w314 -> [w372] mode=indexing
          tunnel: [w358] -> w313 mode=indexing
          tunnel: [errorcluster {"status"=FALSE, "code"=0, "source"=""} ("error in (no error)")] -> w310
          n188 = Index Array(array=w372) -> (element #1=w371:dbl, element #2=w370:dbl, element #3=w369:dbl, element #4=w368:dbl, element #5=w367:dbl, element #6=w366:dbl, element #7=w360:dbl, element #8=w365:dbl, element #9=w364:dbl, element #10=w363:dbl)  [unwired: 10 in]
          n189 = Build Array(w371, w370, w369) -> (w362:dbl[])
          n190 = Build Array(w368, w367, w366) -> (w361:dbl[])
          n191 = Build Array(w365, w364, w363) -> (w359:dbl[])
          n192 = Bundle(w362, w361, "Parameter"=w360, w359) -> (w358:cluster{dbl[], dbl[], "Parameter":dbl, dbl[]})  [unwired: 1 in]
        }
        "GBs to Make" <- w313
        n193 = call <vilib>:"Unset Busy.vi"("error in (no error)"=w310) -> ()  [unwired: 10 in, 1 out]
        n194 = Array Size(array=w313) -> (size(s)=→"# of total points":i32)
      }
    }
  }
  n195 = disable-structure shown="Enabled" {
    frame Disabled {
      n196 = Unbundle By Name("Conventional Unit Cell") -> ("Lattice vector a"=w381:dbl[], "Lattice vector b"=w382:dbl[], "Lattice vector c"=w383:dbl[])
      n197 = for {
        tunnel: w381 -> [w388]
        tunnel: w382 -> [w387]
        tunnel: w383 -> [w386]
        tunnel: [w384] -> _ mode=indexing
        n198 = call "Find Repeating Length from Direction.vi"("Tolerance"=0.025, "Lattice vector c"=w386, "Lattice vector b"=w387, "Lattice vector a"=w388) -> ("Repeating Length (A)"=w384:dbl)  [unwired: 7 in]
      }
    }
    frame Enabled {
    }
  }
